vi "Actor Core.vi"(8 "error in":errorcluster, 11 "Changing Panels in":refnum<class "Changing Panels.lvclass">) -> (0 "error out":errorcluster, 3 "Actor out":refnum<class "Actor.lvclass">)   [LabVIEW 2017, in "2. Basic Panel Actors.lvlib" / "Changing Panels.lvclass"]
doc: "The user interface for this panel.\n----\nCopyright: MGI 2016\nAuthor: Derek Trepanier"
uses:
  Changing Panels.lvclass
  panel-manager/Source/MGI-Panel Manager.lvlib
  panel-manager/Source/Panel/Subpanel/Subpanel.vi
  panel-manager/Source/Panel/Subpanel/Subpanel.lvclass
  Description Panel/Description Panel.lvclass
  panel-actors/Source/Panel Actor/Panel Actor.lvclass
  <vilib>/ActorFramework/Stop Msg/Stop Msg.lvclass
  Panel/Sample Panel.lvclass
  <vilib>/ActorFramework/Message Enqueuer/Message Enqueuer.lvclass
  panel-manager/Source/Panel/Window/Window.vi
  panel-manager/Source/Panel/Window/Window.lvclass
  panel-manager/Source/Window Position/Reference Position/Ref Display/Ref Display.vi
  panel-manager/Source/Window Position/Reference Position/Ref Display/Ref Display.lvclass
  panel-manager/Source/Window Position/Reference Position/Size/Reference Size/Reference Size.vi
  panel-manager/Source/Window Position/Reference Position/Size/Reference Size/Reference Size.lvclass
  D:/test/LabView_PanelManager/panel-manager/Source/Panel/Panel.lvclass
  panel-actors/Source/Panel Actor Messages/Change Panel Msg/Change Panel Msg.lvclass
  panel-actors/Source/Panel Actor Messages/Show Panel Msg/Show Panel Msg.lvclass
  D:/test/LabView_PanelManager/panel-actors/Source/Panel Actor/Panel Actor.lvclass
  D:/test/LabView_PanelManager/panel-manager/Source/Window Position/Reference Position/Size/Size.lvclass
  D:/test/LabView_PanelManager/panel-manager/Source/Window Position/Reference Position/Reference Position.lvclass
  D:/test/LabView_PanelManager/panel-manager/Source/Window Position/Window Position.lvclass
  <vilib>/ActorFramework/Actor/Actor.lvclass
panel:
  in  "Items":i32(listbox)
  in  "New Item":bool
  in  "Undock":bool
  # "Select an item to the left to view its panel"
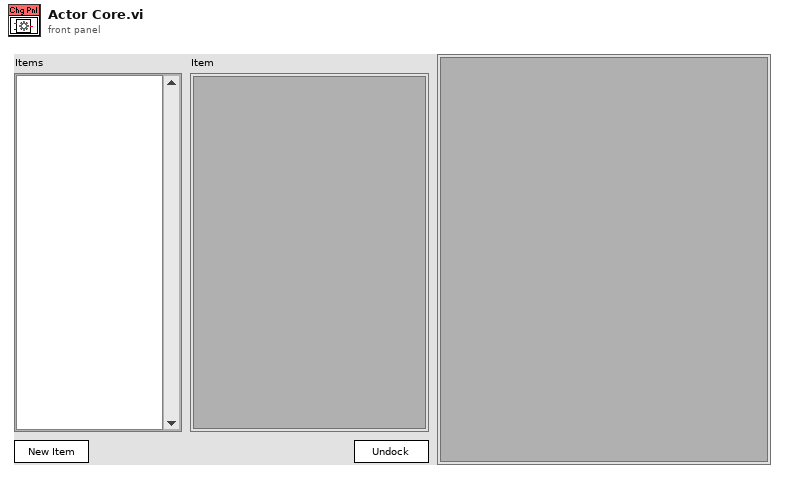
[diagram p1: front panel]
types:
  T1 = enum8{"Enabled", "Disabled", "Disabled and Grayed Out"}
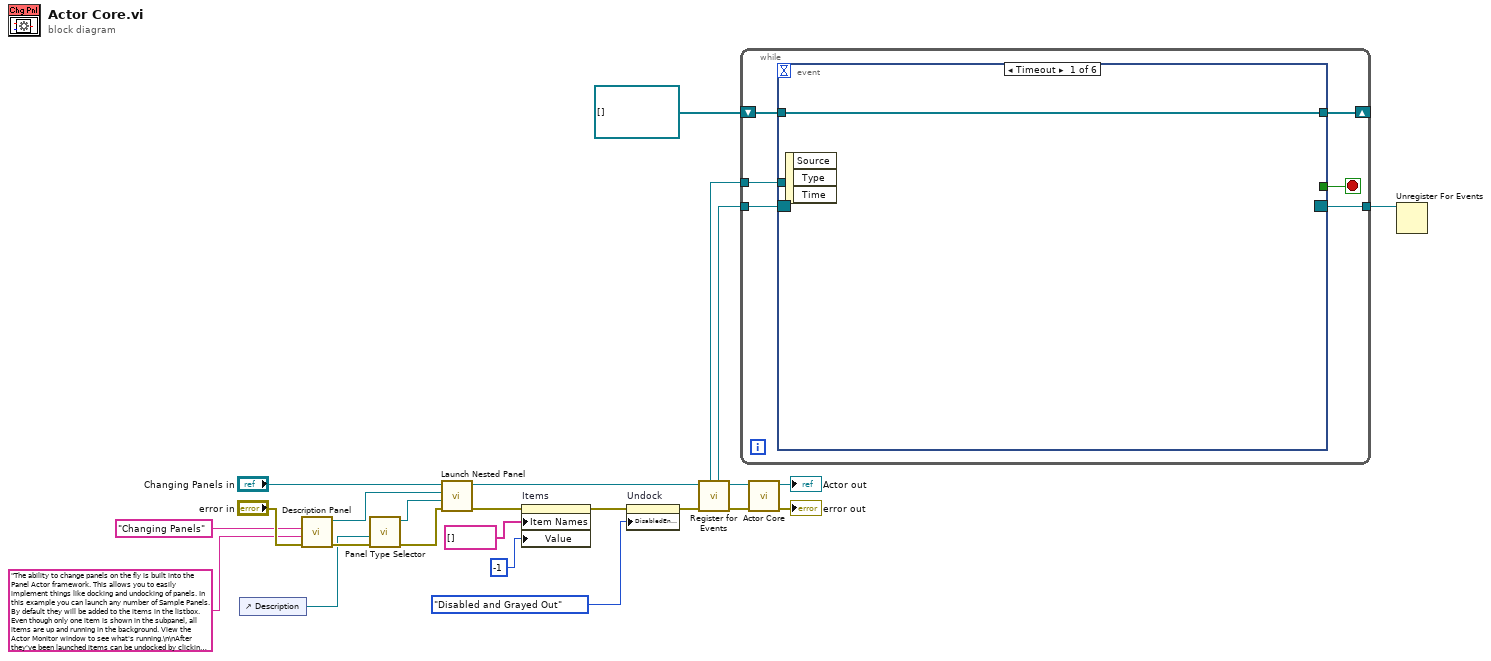
[diagram p0: block diagram]
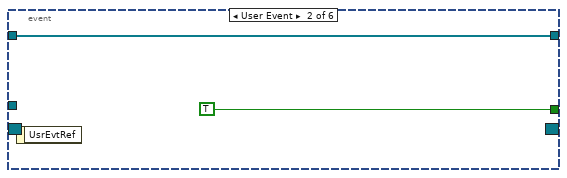
[diagram p2: hidden frame]
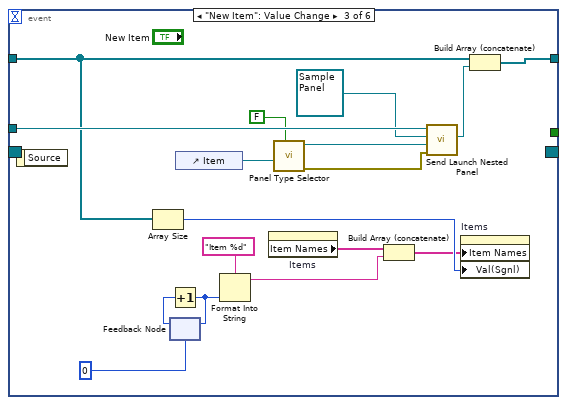
[diagram p3: hidden frame]
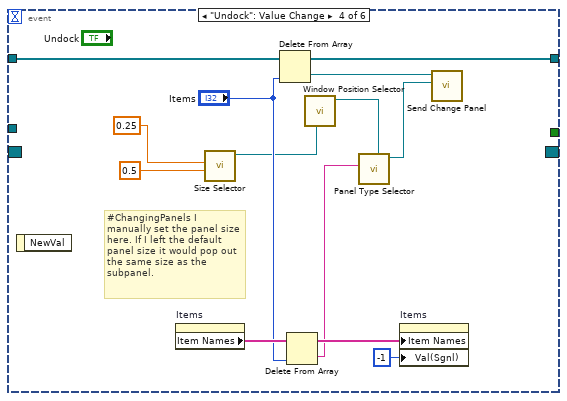
[diagram p4: hidden frame]
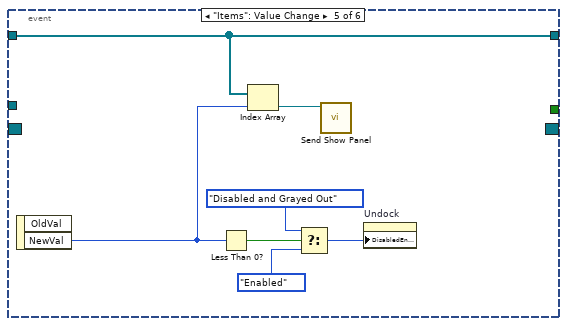
[diagram p5: hidden frame]
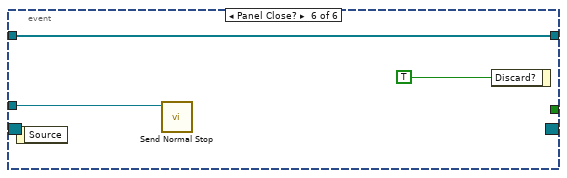
[diagram p6: hidden frame]
diagram:
  n1 = control-ref of="Description"() -> (w2:refnum<vi>)
  n2 = call "Description Panel.vi"("error in (no error)"="error in", "Description"="The ability to change panels on the fly is built into the Panel Actor framework. This allows you to easily implement things like docking and undocking of panels. In this example you can launch any number of Sample Panels. By default they will be added to the items in the listbox. Even though only one item is shown in the subpanel, all items are up and running in the background. View the Actor Monitor window to see what's running.\n\nAfter they've been launched items can be undocked by clicking the \"Undock\" button. This will send a \"Change Panel\" message to the panel actor with the new Window Panel object to use.\n\nThe Sample Panel Actor logs all panel events it encounters. Notice how the events that it receives when the panel changes. First it gets a Panel <b>Closed</b> Event. This is because the Subpanel Object is being closed. Next it gets a Panel <b>Initialized</b> Event. This is because the window was initialized. Finally it gets a Panel <b>Shown</b> Event.\n\nSee the #ChangingPanels bookmark for more info." ("Description Title"), "Description Title"="Changing Panels") -> ("error out"=w21:errorcluster, "Description Panel out"=w18:refnum<class "Description Panel.lvclass">)  [unwired: 7 in]
  n3 = call-poly "Panel Type Selector.vi"("Error In"=w21, "Sub Panel"=w2) -> ("Error Out"=w19:errorcluster, "Subpanel Out"=w20:refnum<class "Subpanel.lvclass">)  [unwired: 8 in]
  n4 = call "Launch Nested Panel.vi"("error in (no error)"=w19, "Panel"=w20, "Nested Panel Actor"=w18, "Panel Actor in"="Changing Panels in") -> ("error out"=w8:errorcluster, "Panel Actor out"=w13:refnum<class "Changing Panels.lvclass">)  [unwired: 4 in, 2 out]
  n5 = property on="Items" class="LstBox (strict)"(error in=w8, "Item Names"=string[] [], "Value"=-1 ("Items")) -> (error out=w5:errorcluster)  [unwired: 1 in, 1 out]
  n6 = property on="Undock" class="Bool"(error in=w5, "DisabledEnum"=T1."Disabled and Grayed Out" ("Disabled")) -> (error out=w4:errorcluster)  [unwired: 1 in, 1 out]
  n7 = call "Register for Events.vi"("Error In"=w4, "Panel Actor in"=w13) -> ("Error Out"=w14:errorcluster, "Panel Actor out"=w12:refnum<class "Changing Panels.lvclass">, "Pnl Actor"=w11:refnum<event-registration>, "Self Enqueuer"=w10:refnum<class "Message Enqueuer.lvclass">)  [unwired: 5 in, 1 out]
  n8 = while {
    tunnel: w11 -> [w30]
    tunnel: w10 -> [w28]
    shift-right: [w26] -> _
    shift-left: refnum<class "Message Enqueuer.lvclass">[] [] -> [w27]
    tunnel: [w25] -> w1
    stop <- w29 stop-if-true
    n9 = event shown="[0] Timeout" {
      selector: w30 -> [_ _ _ _ _ _]
      dyn-events: [_ _ _ _ _ _] -> w25
      timeout: _ -> [_ _ _ _ _ _]
      tunnel: [_ TRUE _ _ _ _] -> w29
      tunnel: w28 -> [_ _ w48 _ _ w72]
      tunnel: w27 -> [w31 w32 w44 w63 w66 w71]
      tunnel: [w31 w32 w49 w62 w66 w71] -> w26
      event Timeout {
        n10 = event-data() -> ()  [unwired: 1 in, 3 out]
      }
      event User Event {
        n11 = event-data() -> ()  [unwired: 1 in, 1 out]
      }
      event "New Item": Value Change {
        n12 = event-data() -> ()  [unwired: 1 in, 1 out]
        n13 = Array Size(array=w44) -> (size(s)=w39:i32)
        n14 = feedback #1(0) -> (w42:i32)
        n15 = Increment(x=w42) -> (x+1=w40:i32)
        n16 = feedback-in #1(w40) -> ()
        n17 = control-ref of="Item"() -> (w50:refnum<vi>)
        n18 = Format Into String(format string="Item %d", w40) -> (resulting string=w36:string)  [unwired: 2 in, 1 out]
        n19 = property on="Items" class="LstBox (strict)"() -> ("Item Names"=w37:string[])  [unwired: 2 in, 2 out]
        n20 = call-poly "Panel Type Selector.vi"("Autoshow? (T)"=FALSE, "Sub Panel"=w50) -> ("Error Out"=w45:errorcluster, "Subpanel Out"=w46:refnum<class "Subpanel.lvclass">)  [unwired: 8 in]
        n21 = Build Array (concatenate)(w37, w36) -> (w38:string[])
        n22 = call "Send Launch Nested Panel.vi"("Error In"=w45, "Panel"=w46, "Nested Panel Actor"=refnum<class "Sample Panel.lvclass"> refnum ("2. Basic Panel Actors.lvlib:Sample Panel.lvclass"), "Self Enqueuer in"=w48) -> ("Nested Actor's Enqueuer"=w47:refnum<class "Message Enqueuer.lvclass">)  [unwired: 5 in, 2 out]
        n23 = property on="Items" class="LstBox (strict)"("Item Names"=w38, "Val(Sgnl)"=w39) -> ()  [unwired: 2 in, 2 out]
        n24 = Build Array (concatenate)(w44, w47) -> (w49:refnum<class "Message Enqueuer.lvclass">[])
      }
      event "Undock": Value Change {
        # "#ChangingPanels I manually set the panel size here. If I left the default panel size it would pop out the same size as the subpanel."
        n25 = event-data() -> ()  [unwired: 1 in, 1 out]
        n26 = property on="Items" class="LstBox (strict)"() -> ("Item Names"=w57:string[])  [unwired: 2 in, 2 out]
        n27 = call-poly "Size Selector.vi"("Height Scale"=0.5 ("Width Scale"), "Width Scale"=0.25) -> ("Static Out"=w53:refnum<class "Reference Size.lvclass">)  [unwired: 8 in, 1 out]
        n28 = Delete From Array(array=w63, index="Items") -> (deleted portion=w61:refnum<class "Message Enqueuer.lvclass">, array with subset deleted=w62:refnum<class "Message Enqueuer.lvclass">[])  [unwired: 1 in]
        n29 = Delete From Array(array=w57, index="Items") -> (deleted portion=w54:string, array with subset deleted=w56:string[])  [unwired: 1 in]
        n30 = call-poly "Window Position Selector.vi"("Size"=w53) -> ("Ref Display out"=w59:refnum<class "Ref Display.lvclass">)  [unwired: 9 in, 1 out]
        n31 = call-poly "Panel Type Selector.vi"("Window Position"=w59, "Default Title"=w54) -> ("Window out"=w60:refnum<class "Window.lvclass">)  [unwired: 8 in, 1 out]
        n32 = property on="Items" class="LstBox (strict)"("Item Names"=w56, "Val(Sgnl)"=-1 ("Value (Signaling)")) -> ()  [unwired: 2 in, 2 out]
        n33 = call "Send Change Panel.vi"("New Panel"=w60, "Message Enqueuer in"=w61) -> ()  [unwired: 8 in, 2 out]
      }
      event "Items": Value Change {
        n34 = event-data() -> ("NewVal"=w65:i32)  [unwired: 1 in, 1 out]
        n35 = Less Than 0?(x=w65) -> (x < 0?=w70:bool)
        n36 = Index Array(array=w66, index=w65) -> (element=w64:refnum<class "Message Enqueuer.lvclass">)
        n37 = Select(t=T1."Disabled and Grayed Out" ("Disabled"), s=w70, f=T1."Enabled" ("Disabled")) -> (s? t:f=w67:T1)
        n38 = call "Send Show Panel.vi"("Message Enqueuer in"=w64) -> ()  [unwired: 9 in, 2 out]
        n39 = property on="Undock" class="Bool"("DisabledEnum"=w67) -> ()  [unwired: 2 in, 2 out]
      }
      event Panel Close? {
        n40 = event-data() -> ()  [unwired: 1 in, 1 out]
        n41 = call <vilib>:"Send Normal Stop.vi"("Message Enqueuer"=w72) -> ()  [unwired: 10 in, 1 out]
        n42 = event-data("Discard?"=TRUE) -> ()  [unwired: 1 in, 1 out]
      }
    }
  }
  n43 = call-parent "Actor Core.vi"("error in"=w14, "Panel Actor in"=w12) -> ("error out"=→"error out":errorcluster, "Actor out"=→"Actor out":refnum<class "Actor.lvclass">)  [unwired: 8 in]
  n44 = Unregister For Events(event registration refnum=w1) -> ()  [unwired: 1 in, 1 out]
